vi "Unit Test.vi"() -> ()   [LabVIEW 2019, in "ADLINK Motion Card.lvlib"]
uses:
  ADLINK Motion Card.lvlib
  User Event/Controls/UE Abort Action.ctl
panel:
  out "Y Arrived?":bool
  out "X Arrived?":bool
  in  "stop":bool
  in  "Y Move":bool
  in  "X Move":bool
  in  "Y Acceleration":dbl
  in  "X Acceleration":dbl
  in  "Y Velocity":dbl
  in  "X Velocity":dbl
  out "Y Current Position":dbl
  out "X Current Position":dbl
  in  "Y Target Position":dbl
  in  "X Target Position":dbl
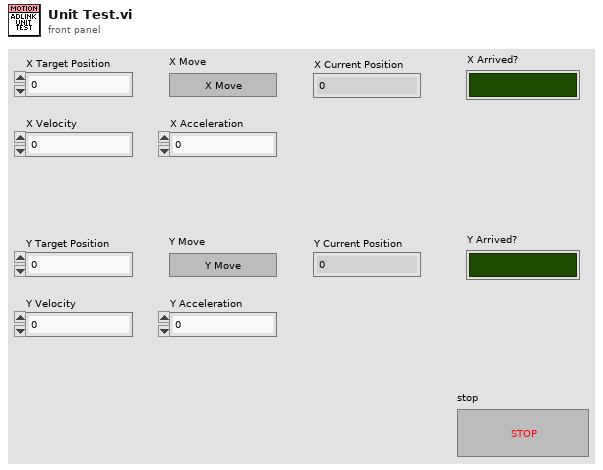
[diagram p1: front panel]
types:
  T1 = typedef "UE Abort Action.ctl" = enum16{"Create", "Get", "Destroy"}
  T2 = typedef "ADLINK Motion Card.lvlib/SEQ Data.ctl" = cluster{"Current Position":dbl, "Target Position":dbl, "Velocity":dbl, "Acceleration":dbl, "Arrived?":bool, "data value reference":refnum<data-value>, "VI Refnum":refnum<vi>}
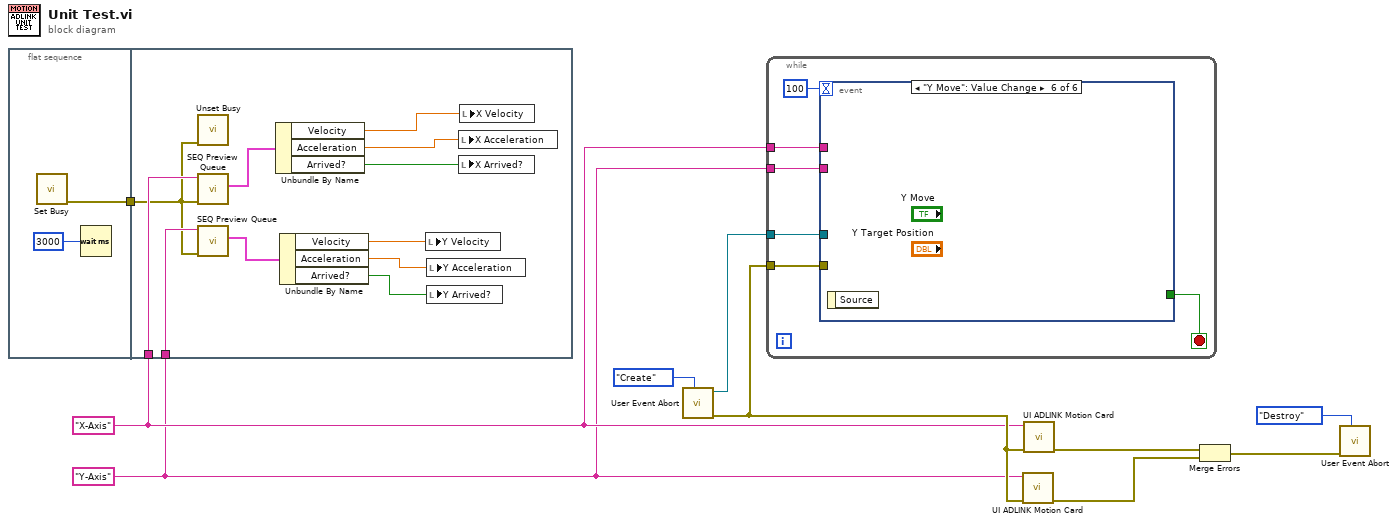
[diagram p0: block diagram]
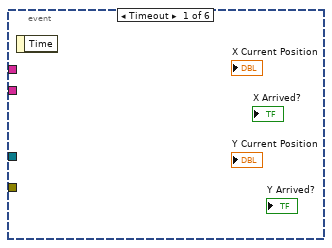
[diagram p2: hidden frame]
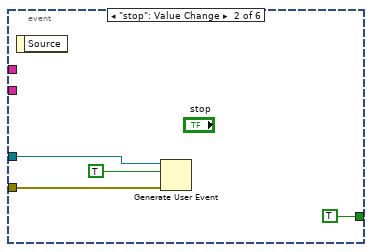
[diagram p3: hidden frame]
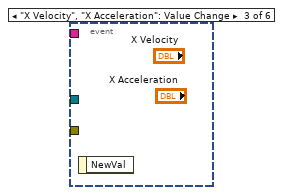
[diagram p4: hidden frame]
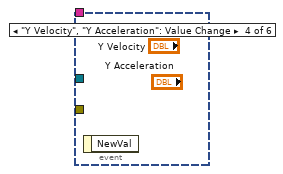
[diagram p5: hidden frame]
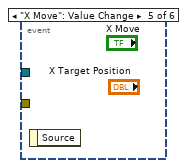
[diagram p6: hidden frame]
diagram:
  w4 = "Y-Axis" ("Module Name")
  w5 = "X-Axis" ("Module Name")
  n1 = flat-sequence {
    tunnel: [w11] -> w10
    tunnel: w10 -> [w17]
    tunnel: w5 -> [w23]
    tunnel: w4 -> [w22]
    frame #0 {
      n2 = call <vilib>:"Set Busy.vi"() -> ("error out"=w11:errorcluster)  [unwired: 10 in, 1 out]
      n3 = Wait (ms)(milliseconds to wait=u32 3000) -> ()  [unwired: 1 out]
    }
    frame #1 {
      n4 = call <vilib>:"Unset Busy.vi"("error in (no error)"=w17) -> ()  [unwired: 10 in, 1 out]
      n5 = call "SEQ Preview Queue.vi"("error in (no error)"=w17, "Queue Name"=w23) -> ("Setting"=w21:T2)  [unwired: 8 in, 1 out]
      n6 = call "SEQ Preview Queue.vi"("error in (no error)"=w17, "Queue Name"=w22) -> ("Setting"=w16:T2)  [unwired: 8 in, 1 out]
      n7 = Unbundle By Name(w21) -> ("Velocity"=w18:dbl, "Acceleration"=w19:dbl, "Arrived?"=w20:bool)
      n8 = Unbundle By Name(w16) -> ("Velocity"=w15:dbl, "Acceleration"=w14:dbl, "Arrived?"=w13:bool)
      n9 = local write "Y Velocity"(w15) -> ()
      n10 = local write "Y Acceleration"(w14) -> ()
      n11 = local write "Y Arrived?"(w13) -> ()
      n12 = local write "X Acceleration"(w19) -> ()
      n13 = local write "X Arrived?"(w20) -> ()
      n14 = local write "X Velocity"(w18) -> ()
    }
  }
  n15 = call "User Event Abort.vi"("Action"=UE_Abort_Action."Create") -> ("Error Out"=w6:errorcluster, "User Event Out"=w7:refnum<user-event>)  [unwired: 9 in]
  n16 = while {
    tunnel: w7 -> [w28]
    tunnel: w6 -> [w27]
    tunnel: w5 -> [w26]
    tunnel: w4 -> [w25]
    stop <- w29 stop-if-true
    n17 = event shown="[5] \"Y Move\": Value Change" {
      selector: _ -> [_ _ _ _ _ _]
      dyn-events: _ -> [_ _ _ _ _ _]
      timeout: 100 -> [_ _ _ _ _ _]
      tunnel: [_ TRUE _ _ _ _] -> w29
      tunnel: w28 -> [_ w32 _ _ _ _]
      tunnel: w27 -> [_ w31 _ _ _ _]
      tunnel: w26 -> [_ _ _ _ _ _]
      tunnel: w25 -> [_ _ _ _ _ _]
      event Timeout {
        n18 = event-data() -> ()  [unwired: 1 in, 1 out]
      }
      event "stop": Value Change {
        n19 = event-data() -> ()  [unwired: 1 in, 1 out]
        n20 = Generate User Event(user event=w32, event data cluster=TRUE ("event data"), error in=w31) -> ()  [unwired: 1 in, 2 out]
      }
      event "X Velocity", "X Acceleration": Value Change {
        n21 = event-data() -> ()  [unwired: 1 in, 1 out]
      }
      event "Y Velocity", "Y Acceleration": Value Change {
        n22 = event-data() -> ()  [unwired: 1 in, 1 out]
      }
      event "X Move": Value Change {
        n23 = event-data() -> ()  [unwired: 1 in, 1 out]
      }
      event "Y Move": Value Change {
        n24 = event-data() -> ()  [unwired: 1 in, 1 out]
      }
    }
  }
  n25 = call "UI ADLINK Motion Card.vi"("error in (no error)"=w6, "Module Name"=w4) -> ("error out"=w2:errorcluster)  [unwired: 9 in]
  n26 = call "UI ADLINK Motion Card.vi"("error in (no error)"=w6, "Module Name"=w5) -> ("error out"=w3:errorcluster)  [unwired: 9 in]
  n27 = Merge Errors(w3, w2) -> (w1:errorcluster)
  n28 = call "User Event Abort.vi"("Action"=UE_Abort_Action."Destroy", "Error In"=w1) -> ()  [unwired: 8 in, 2 out]
